vi "Start Logic-Mode dependent case 2.vi"(6 "Case name string":string, 8 "error in (no error)":errorcluster, 9 "cancelled":bool, 10 "UI queue":refnum<queue>, 11 "Acq. queue in":refnum<queue>) -> (0 "error out":errorcluster, 3 "Acq. queue out":refnum<queue>)   [LabVIEW 2017]
uses:
  Queue/Message Queue/Typedefs/Message Cluster.ctl
  Typedefs/Read Write Enum.ctl
  Typedefs/Top level VI states.ctl
  Global Variables/gl_UI Ctrl Refs.vi
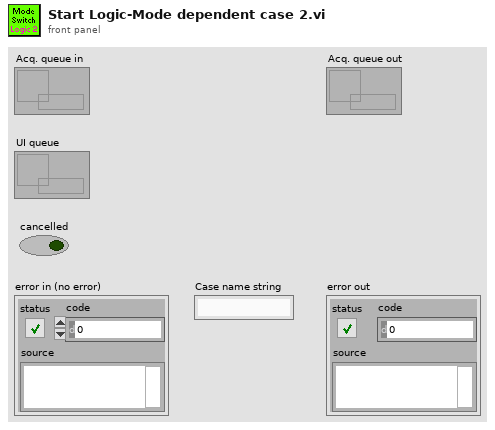
[diagram p1: front panel]
types:
  T1 = typedef "Read Write Enum.ctl" = enum16{"Read", "Write"}
  T2 = typedef "Top level VI states.ctl" = enum16{"None", "Initialise UI", "<STACK PROTOCOL STATES>", "AOL Zstack-START", "AOL Zstack-STOP", "Motor Zstack-START", "Motor Zstack-STOP", "<ACQUISITION PROTOCOL STATES> ", "Functional Acquisition-START", "Functional Acquisition-STOP", "Single Plane Acquisition-START", "Single Plane Acquisition-STOP", "Volume Acquisition-START", "Volume Acquisition-STOP", "<LIVE IMAGING PROTOCOL STATES>", "Live Imaging-START", "Live Imaging-STOP", "Live Plane Imaging-START", "Live Plane Imaging-STOP", "Live Volume Imaging-START", "Live Volume Imaging-STOP", "<MOVEMENT CORRECTION PROTOCOL STATES>", "EXIT"}
  T3 = typedef "UI ctrl refs cluster.ctl" = cluster{"Top level VI path":path, "Top level VI ref":refnum<vi>, "User menu ref":refnum<k9>, "Sub Panel control":refnum<vi>, "Imaging Param Tab":refnum<vi>, "Occurrence-Start drivers":refnum<k4>, "Occurrence-Speed logging initialised":refnum<k4>, "Occurrence-XYZ stage initialised":refnum<k4>, "Exit button":refnum<vi>, "Status ind":refnum<vi>, "Set as origin":refnum<vi>, "Speed Logging":refnum<vi>, "Time Lapse":refnum<vi>, "Live Imaging":refnum<vi>, "AOL Z Stack":refnum<vi>, "Motor Z Stack":refnum<vi>, "Funct Acq button":refnum<vi>, "Hard Shutter":refnum<vi>, "Virtual Shutter":refnum<vi>, "Laser Power":refnum<vi>, "AOL Mode":refnum<vi>, "Frame Size":refnum<vi>, "Field of View":refnum<vi>, "Dwell Time":refnum<vi>, "Zoom":refnum<vi>, "AOL Z":refnum<vi>, "Objective":refnum<vi>, "Axis":refnum<vi>, "Paths & Names":refnum<vi>, "Experiment folder path (ind.)":refnum<vi>, "Last State (Ind.)":refnum<vi>, "Averages":refnum<vi>, "Angle (degrees)":refnum<vi>, "X centre":refnum<vi>, "Y centre":refnum<vi>, "Plane Mode":refnum<vi>, "# Planes":refnum<vi>, "Z Start":refnum<vi>, "Z Stop":refnum<vi>, "Z Step":refnum<vi>, "PMT 1":refnum<vi>, "PMT 2":refnum<vi>, "Stage XYZ Position":refnum<vi>, "Pockels@Z Start":refnum<vi>, "Pockels@Z Stop":refnum<vi>, "Obtain Z Start":refnum<vi>, "Obtain Z Stop":refnum<vi>, "Live stim.trig.period":refnum<vi>, "Live stim.trig.enable":refnum<vi>, "XY Stage Move":refnum<vi>, "Funct. Acq. Pockels Modulation":refnum<vi>, "Enable Video Recording":refnum<vi>, "Video Record-Live Imaging":refnum<vi>, "Video Record-Funct acq":refnum<vi>, "AOL Z-stack Chirps Ready (ind)":refnum<vi>, "Target time between mov.cor. ref triggers (ms)":refnum<vi>, "Center freq ind (nm)":refnum<vi>, "Pickup mode (ind)":refnum<vi>, "Logging queue (ind)":refnum<vi>, "Back aperture power (ind.)":refnum<vi>, "Power after objective (ind.)":refnum<vi>, "Switch user":refnum<vi>, "Ls1 Conn. Status":refnum<vi>, "Ls1Tuning Status":refnum<vi>, "Ls1 Faults":refnum<vi>, "Ls1 Connection":refnum<vi>, "Ls1 Mode":refnum<vi>, "Ls1 POWER [mW]":refnum<vi>, "Ls1Shutter":refnum<vi>, "Ls1 Wavelength":refnum<vi>, "Ls1 Note":refnum<vi>, "Ls1 Confirm Wav":refnum<vi>, "Ls1 PreChrp Prism1":refnum<vi>, "Ls1 PreChrp Prism2":refnum<vi>, "Ls1 wav top Ind":refnum<vi>, "Ls1 power top Ind":refnum<vi>, "Ls1 Pump peak Hold":refnum<vi>, "Ls1 Status Ind":refnum<vi>, "Ls1 wav cancel":refnum<vi>, "Experiment Type":refnum<vi>, "Biology Information":refnum<vi>}
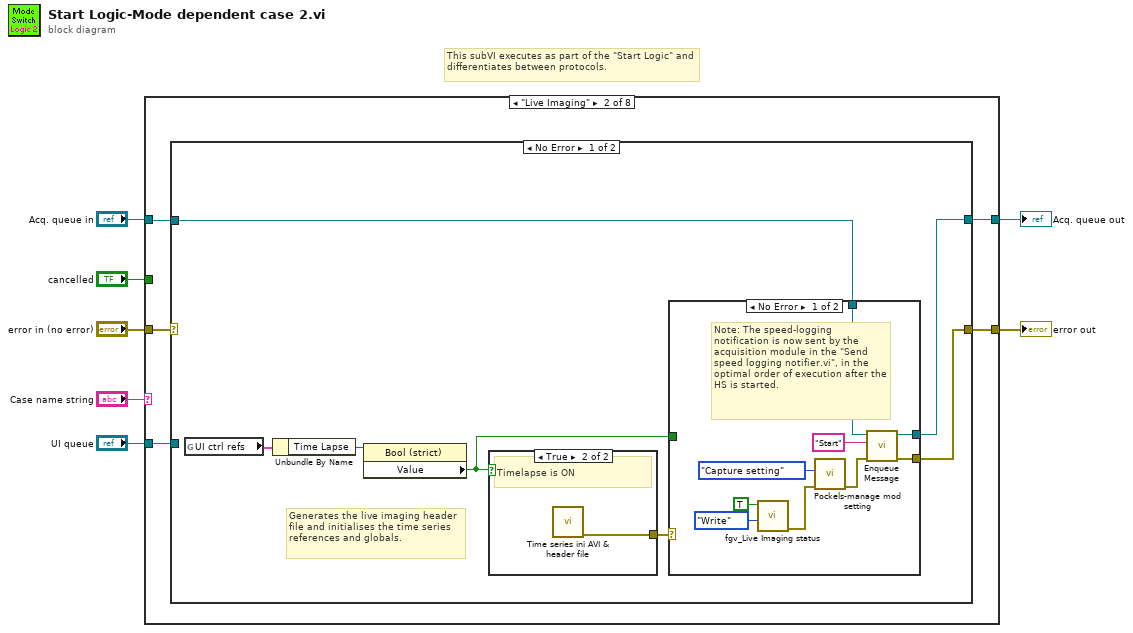
[diagram p0: block diagram]
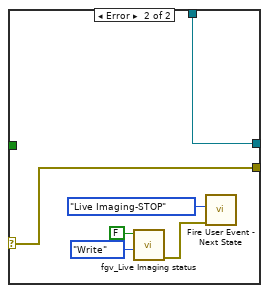
[diagram p3: hidden frame]
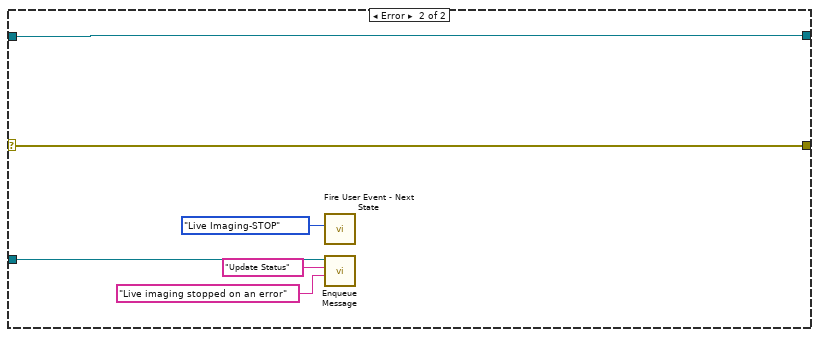
[diagram p5: hidden frame]
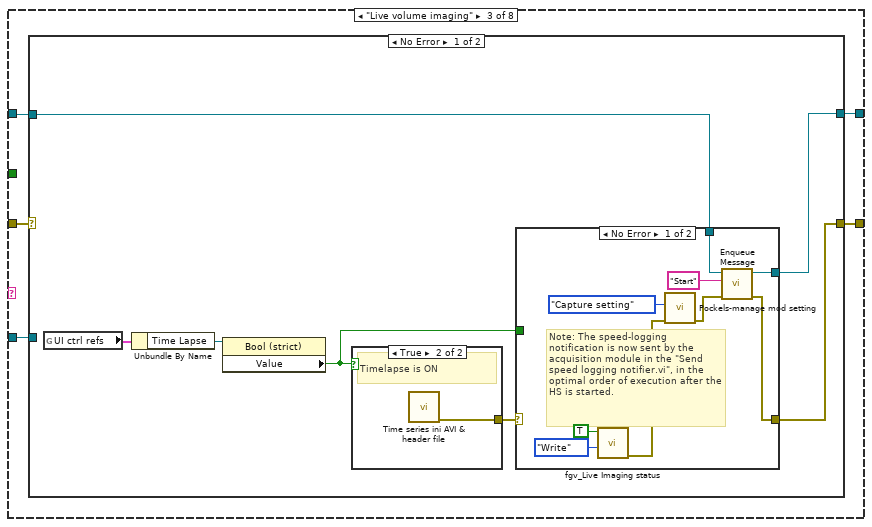
[diagram p6: hidden frame]
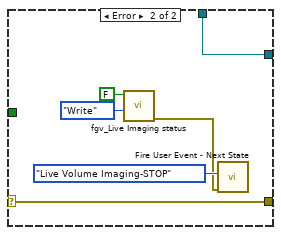
[diagram p7: hidden frame]
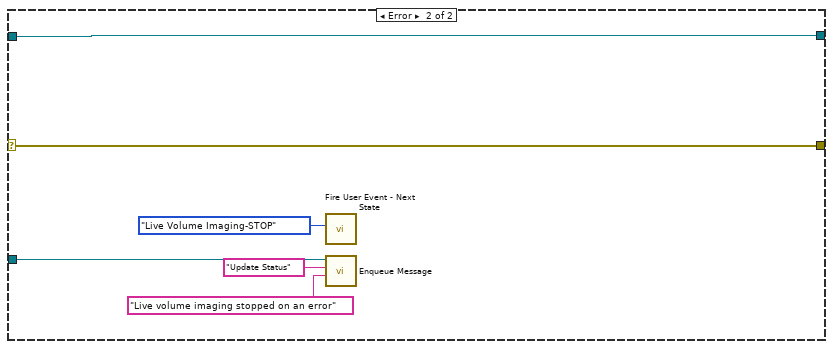
[diagram p9: hidden frame]
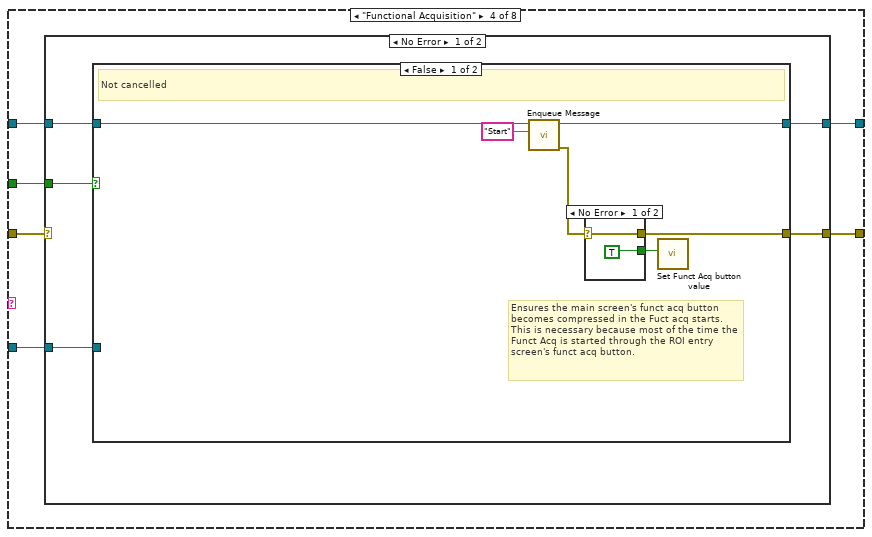
[diagram p10: hidden frame]
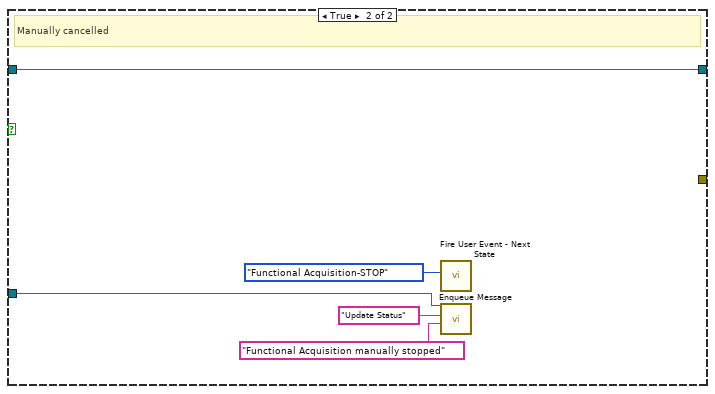
[diagram p12: hidden frame]
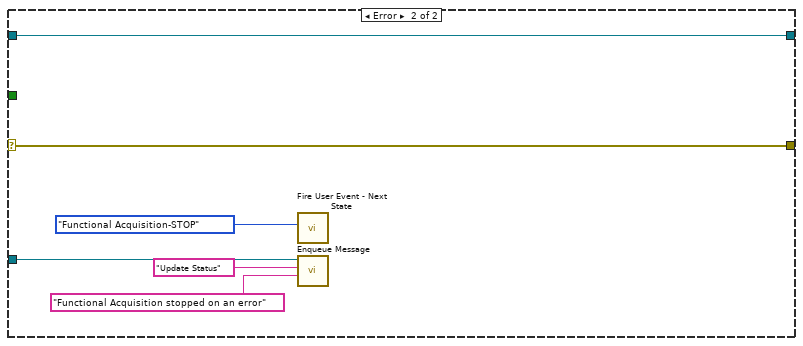
[diagram p13: hidden frame]
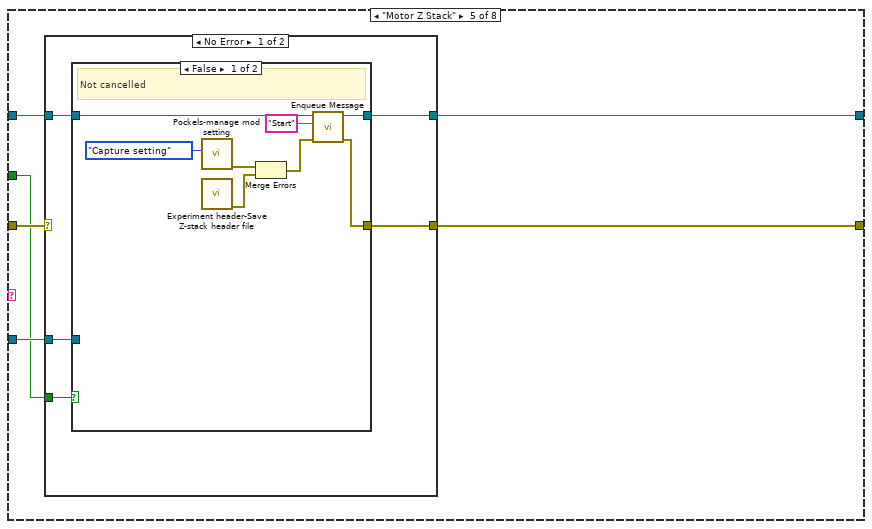
[diagram p14: hidden frame]
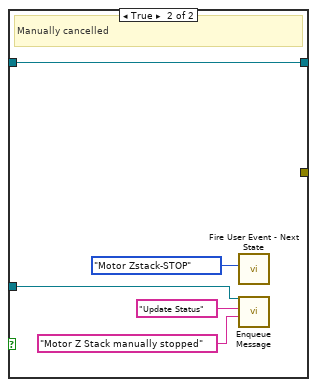
[diagram p15: hidden frame]
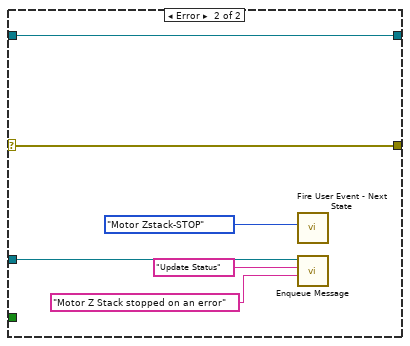
[diagram p16: hidden frame]
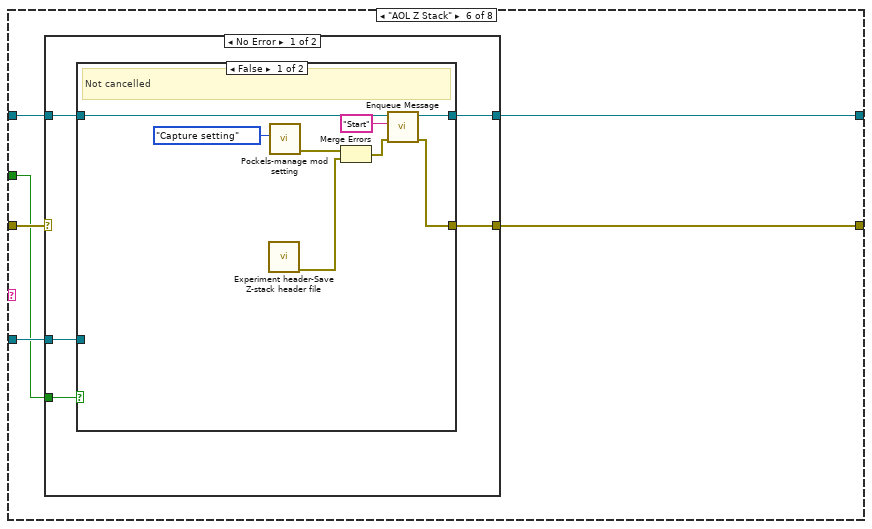
[diagram p17: hidden frame]
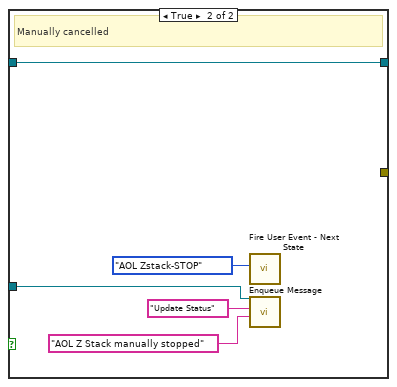
[diagram p18: hidden frame]
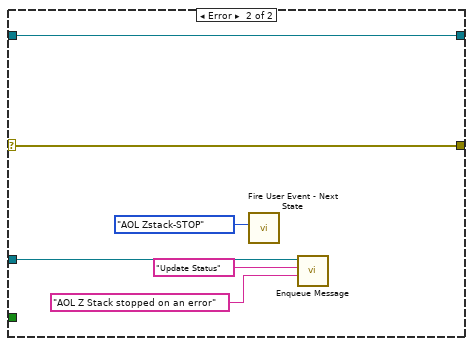
[diagram p19: hidden frame]
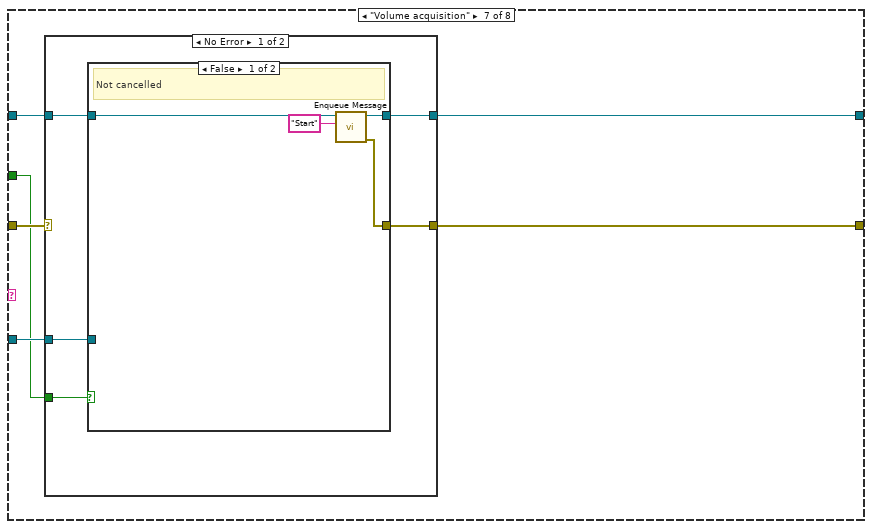
[diagram p20: hidden frame]
diagram:
  # "This subVI executes as part of the \"Start Logic\" and differentiates between protocols."
  n1 = case shown="\"Live Imaging\"" "Case name string" {
    tunnel: [w9 w14 w48 w80 w111 w141 w171 w197] -> w1
    tunnel: "error in (no error)" -> [w9 w11 w45 w81 w112 w142 w172 w198]
    tunnel: [w8 w12 w46 w83 w114 w144 w174 w200] -> w3
    tunnel: "Acq. queue in" -> [w8 w13 w47 w82 w113 w143 w173 w199]
    tunnel: "UI queue" -> [_ w10 w44 w79 w110 w140 w170 w196]
    tunnel: "cancelled" -> [_ _ _ w78 w109 w139 w169 w195]
    frame Default {
    }
    frame "Live Imaging" {
      n2 = case shown="No Error" w11 {
        selector: w11 -> [_ w43]
        tunnel: [w16 w43] -> w14
        tunnel: w13 -> [w18 w42]
        tunnel: [w17 w42] -> w12
        tunnel: w10 -> [_ w38]
        frame No Error {
          # "Generates the live imaging header file and initialises the time series references and globals."
          n3 = global read "gl_UI Ctrl Refs.vi" "UI ctrl refs"() -> (w15:T3)
          n4 = Unbundle By Name(w15) -> ("Time Lapse"=w21:refnum<vi>)
          n5 = property class="Bool (strict)"(reference=w21) -> ("Value"=w19:bool)  [unwired: 1 in, 2 out]
          n6 = case shown="True" w19 {
            tunnel: [_ w37] -> w20
            frame False {
              # "Timelapse is OFF"
            }
            frame True {
              # "Timelapse is ON"
              n7 = call "Time series ini AVI & header file.vi"() -> ("error out"=w37:errorcluster)  [unwired: 11 in]
            }
          }
          n8 = case shown="No Error" w20 {
            selector: w20 -> [_ w34]
            tunnel: w19 -> [_ _]
            tunnel: w18 -> [w27 w35]
            tunnel: [w29 w35] -> w17
            tunnel: [w28 w34] -> w16
            frame No Error {
              # "Note: The speed-logging notification is now sent by the acquisition module in the \"Send speed logging notifier.vi\", in the optimal order of execution after the HS is started."
              n9 = call "fgv_Live Imaging status.vi"("Function"=Read_Write_Enum."Write", "Live Imaging?"=TRUE ("Timelapse?")) -> ("error out"=w22:errorcluster)  [unwired: 8 in, 1 out]
              n10 = call "Pockels-manage mod setting.vi"("error in (no error)"=w22, "Function"=enum16{"Capture setting", "Re-apply setting"}."Capture setting") -> ("error out"=w26:errorcluster)  [unwired: 9 in]
              n11 = call "Enqueue Message.vi"("error in (no error)"=w26, "Message"="Start", "Queue"=w27) -> ("error out"=w28:errorcluster, "Queue out"=w29:refnum<queue>)  [unwired: 7 in]
            }
            frame Error {
              n12 = call "fgv_Live Imaging status.vi"("Function"=Read_Write_Enum."Write", "Live Imaging?"=FALSE ("Timelapse?")) -> ("error out"=w31:errorcluster)  [unwired: 8 in, 1 out]
              n13 = call "Fire User Event - Next State.vi"("Error In"=w31, "\"UI Handler loop\" case to execute"=Top_level_VI_states."Live Imaging-STOP" ("event data / imaging mode")) -> ()  [unwired: 9 in, 1 out]
            }
          }
        }
        frame Error {
          n14 = call "Fire User Event - Next State.vi"("\"UI Handler loop\" case to execute"=Top_level_VI_states."Live Imaging-STOP" ("event data / imaging mode")) -> ()  [unwired: 10 in, 1 out]
          n15 = call "Enqueue Message.vi"("Message Data"="Live imaging stopped on an error" ("Acquiring and Logging..."), "Message"="Update Status", "Queue"=w38) -> ()  [unwired: 7 in, 2 out]
        }
      }
    }
    frame "Live volume imaging" {
      n16 = case shown="No Error" w45 {
        selector: w45 -> [_ w77]
        tunnel: [w52 w77] -> w48
        tunnel: w47 -> [w51 w76]
        tunnel: [w50 w76] -> w46
        tunnel: w44 -> [_ w73]
        frame No Error {
          n17 = global read "gl_UI Ctrl Refs.vi" "UI ctrl refs"() -> (w49:T3)
          n18 = Unbundle By Name(w49) -> ("Time Lapse"=w55:refnum<vi>)
          n19 = property class="Bool (strict)"(reference=w55) -> ("Value"=w53:bool)  [unwired: 1 in, 2 out]
          n20 = case shown="True" w53 {
            tunnel: [_ w71] -> w54
            frame False {
              # "Timelapse is OFF"
            }
            frame True {
              # "Timelapse is ON"
              n21 = call "Time series ini AVI & header file.vi"() -> ("error out"=w71:errorcluster)  [unwired: 11 in]
            }
          }
          n22 = case shown="No Error" w54 {
            selector: w54 -> [_ w70]
            tunnel: [w63 w70] -> w52
            tunnel: w53 -> [_ _]
            tunnel: w51 -> [w62 w68]
            tunnel: [w61 w68] -> w50
            frame No Error {
              # "Note: The speed-logging notification is now sent by the acquisition module in the \"Send speed logging notifier.vi\", in the optimal order of execution after the HS is started."
              n23 = call "fgv_Live Imaging status.vi"("Function"=Read_Write_Enum."Write", "Live Imaging?"=TRUE ("Timelapse?")) -> ("error out"=w56:errorcluster)  [unwired: 8 in, 1 out]
              n24 = call "Pockels-manage mod setting.vi"("error in (no error)"=w56, "Function"=enum16{"Capture setting", "Re-apply setting"}."Capture setting") -> ("error out"=w60:errorcluster)  [unwired: 9 in]
              n25 = call "Enqueue Message.vi"("error in (no error)"=w60, "Message"="Start", "Queue"=w62) -> ("error out"=w63:errorcluster, "Queue out"=w61:refnum<queue>)  [unwired: 7 in]
            }
            frame Error {
              n26 = call "fgv_Live Imaging status.vi"("Function"=Read_Write_Enum."Write", "Live Imaging?"=FALSE ("Timelapse?")) -> ("error out"=w65:errorcluster)  [unwired: 8 in, 1 out]
              n27 = call "Fire User Event - Next State.vi"("Error In"=w65, "\"UI Handler loop\" case to execute"=Top_level_VI_states."Live Volume Imaging-STOP" ("event data / imaging mode")) -> ()  [unwired: 9 in, 1 out]
            }
          }
        }
        frame Error {
          n28 = call "Fire User Event - Next State.vi"("\"UI Handler loop\" case to execute"=Top_level_VI_states."Live Volume Imaging-STOP" ("event data / imaging mode")) -> ()  [unwired: 10 in, 1 out]
          n29 = call "Enqueue Message.vi"("Message Data"="Live volume imaging stopped on an error" ("Acquiring and Logging..."), "Message"="Update Status", "Queue"=w73) -> ()  [unwired: 7 in, 2 out]
        }
      }
    }
    frame "Functional Acquisition" {
      n30 = case shown="No Error" w81 {
        selector: w81 -> [_ w107]
        tunnel: [w84 w107] -> w80
        tunnel: [w85 w108] -> w83
        tunnel: w82 -> [w86 w108]
        tunnel: w79 -> [w88 w103]
        tunnel: w78 -> [w87 _]
        frame No Error {
          n31 = case shown="False" w87 {
            tunnel: w88 -> [_ w99]
            tunnel: w86 -> [w93 w98]
            tunnel: [w92 w98] -> w85
            tunnel: [w90 _] -> w84
            frame False {
              # "Ensures the main screen's funct acq button becomes compressed in the Fuct acq starts. This is necessary because most of the time the Funct Acq is started through the ROI entry screen's funct acq button."
              # "Not cancelled"
              n32 = call "Enqueue Message.vi"("Message"="Start", "Queue"=w93) -> ("error out"=w91:errorcluster, "Queue out"=w92:refnum<queue>)  [unwired: 8 in]
              n33 = case shown="No Error" w91 {
                selector: w91 -> [w96 w97]
                tunnel: [w96 w97] -> w90
                tunnel: [TRUE ("Value") _] -> w89
                frame No Error {
                }
                frame Error {
                }
              }
              n34 = call "Set Funct Acq button value.vi"("Functional Acquisition button's new value"=w89) -> ()  [unwired: 10 in, 1 out]
            }
            frame True {
              # "Manually cancelled"
              n35 = call "Fire User Event - Next State.vi"("\"UI Handler loop\" case to execute"=Top_level_VI_states."Functional Acquisition-STOP" ("event data / imaging mode")) -> ()  [unwired: 10 in, 1 out]
              n36 = call "Enqueue Message.vi"("Message Data"="Functional Acquisition manually stopped" ("Acquiring and Logging..."), "Message"="Update Status", "Queue"=w99) -> ()  [unwired: 7 in, 2 out]
            }
          }
        }
        frame Error {
          n37 = call "Fire User Event - Next State.vi"("\"UI Handler loop\" case to execute"=Top_level_VI_states."Functional Acquisition-STOP" ("event data / imaging mode")) -> ()  [unwired: 10 in, 1 out]
          n38 = call "Enqueue Message.vi"("Message Data"="Functional Acquisition stopped on an error" ("Acquiring and Logging..."), "Message"="Update Status", "Queue"=w103) -> ()  [unwired: 7 in, 2 out]
        }
      }
    }
    frame "Motor Z Stack" {
      n39 = case shown="No Error" w112 {
        selector: w112 -> [_ w137]
        tunnel: [w115 w137] -> w111
        tunnel: [w116 w138] -> w114
        tunnel: w113 -> [w117 w138]
        tunnel: w110 -> [w119 w133]
        tunnel: w109 -> [w118 _]
        frame No Error {
          n40 = case shown="False" w118 {
            tunnel: w119 -> [_ w129]
            tunnel: w117 -> [w126 w128]
            tunnel: [w125 w128] -> w116
            tunnel: [w124 _] -> w115
            frame False {
              # "Not cancelled"
              n41 = call "Pockels-manage mod setting.vi"("Function"=enum16{"Capture setting", "Re-apply setting"}."Capture setting") -> ("error out"=w122:errorcluster)  [unwired: 10 in]
              n42 = call "Experiment header-Save Z-stack header file.vi"() -> ("error out"=w121:errorcluster)  [unwired: 11 in]
              n43 = Merge Errors(w122, w121) -> (w120:errorcluster)
              n44 = call "Enqueue Message.vi"("error in (no error)"=w120, "Message"="Start", "Queue"=w126) -> ("error out"=w124:errorcluster, "Queue out"=w125:refnum<queue>)  [unwired: 7 in]
            }
            frame True {
              # "Manually cancelled"
              n45 = call "Fire User Event - Next State.vi"("\"UI Handler loop\" case to execute"=Top_level_VI_states."Motor Zstack-STOP" ("event data / imaging mode")) -> ()  [unwired: 10 in, 1 out]
              n46 = call "Enqueue Message.vi"("Message Data"="Motor Z Stack manually stopped" ("Acquiring and Logging..."), "Message"="Update Status", "Queue"=w129) -> ()  [unwired: 7 in, 2 out]
            }
          }
        }
        frame Error {
          n47 = call "Fire User Event - Next State.vi"("\"UI Handler loop\" case to execute"=Top_level_VI_states."Motor Zstack-STOP" ("event data / imaging mode")) -> ()  [unwired: 10 in, 1 out]
          n48 = call "Enqueue Message.vi"("Message Data"="Motor Z Stack stopped on an error" ("Acquiring and Logging..."), "Message"="Update Status", "Queue"=w133) -> ()  [unwired: 7 in, 2 out]
        }
      }
    }
    frame "AOL Z Stack" {
      n49 = case shown="No Error" w142 {
        selector: w142 -> [_ w167]
        tunnel: [w145 w167] -> w141
        tunnel: [w146 w168] -> w144
        tunnel: w143 -> [w147 w168]
        tunnel: w140 -> [w149 w163]
        tunnel: w139 -> [w148 _]
        frame No Error {
          n50 = case shown="False" w148 {
            tunnel: w149 -> [_ w159]
            tunnel: w147 -> [w156 w158]
            tunnel: [w155 w158] -> w146
            tunnel: [w154 _] -> w145
            frame False {
              # "Not cancelled"
              n51 = call "Experiment header-Save Z-stack header file.vi"() -> ("error out"=w150:errorcluster)  [unwired: 11 in]
              n52 = call "Pockels-manage mod setting.vi"("Function"=enum16{"Capture setting", "Re-apply setting"}."Capture setting") -> ("error out"=w152:errorcluster)  [unwired: 10 in]
              n53 = Merge Errors(w152, w150) -> (w151:errorcluster)
              n54 = call "Enqueue Message.vi"("error in (no error)"=w151, "Message"="Start", "Queue"=w156) -> ("error out"=w154:errorcluster, "Queue out"=w155:refnum<queue>)  [unwired: 7 in]
            }
            frame True {
              # "Manually cancelled"
              n55 = call "Fire User Event - Next State.vi"("\"UI Handler loop\" case to execute"=Top_level_VI_states."AOL Zstack-STOP" ("event data / imaging mode")) -> ()  [unwired: 10 in, 1 out]
              n56 = call "Enqueue Message.vi"("Message Data"="AOL Z Stack manually stopped" ("Acquiring and Logging..."), "Message"="Update Status", "Queue"=w159) -> ()  [unwired: 7 in, 2 out]
            }
          }
        }
        frame Error {
          n57 = call "Fire User Event - Next State.vi"("\"UI Handler loop\" case to execute"=Top_level_VI_states."AOL Zstack-STOP" ("event data / imaging mode")) -> ()  [unwired: 10 in, 1 out]
          n58 = call "Enqueue Message.vi"("Message Data"="AOL Z Stack stopped on an error" ("Acquiring and Logging..."), "Message"="Update Status", "Queue"=w163) -> ()  [unwired: 7 in, 2 out]
        }
      }
    }
    frame "Volume acquisition" {
      n59 = case shown="No Error" w172 {
        selector: w172 -> [_ w193]
        tunnel: [w175 w193] -> w171
        tunnel: [w176 w194] -> w174
        tunnel: w173 -> [w177 w194]
        tunnel: w170 -> [w179 w189]
        tunnel: w169 -> [w178 _]
        frame No Error {
          n60 = case shown="False" w178 {
            tunnel: w179 -> [_ w185]
            tunnel: w177 -> [w182 w184]
            tunnel: [w181 w184] -> w176
            tunnel: [w180 _] -> w175
            frame False {
              # "Not cancelled"
              n61 = call "Enqueue Message.vi"("Message"="Start", "Queue"=w182) -> ("error out"=w180:errorcluster, "Queue out"=w181:refnum<queue>)  [unwired: 8 in]
            }
            frame True {
              # "Manually cancelled"
              n62 = call "Fire User Event - Next State.vi"("\"UI Handler loop\" case to execute"=Top_level_VI_states."Volume Acquisition-STOP" ("event data / imaging mode")) -> ()  [unwired: 10 in, 1 out]
              n63 = call "Enqueue Message.vi"("Message Data"="Volume Acquisition manually stopped" ("Acquiring and Logging..."), "Message"="Update Status", "Queue"=w185) -> ()  [unwired: 7 in, 2 out]
            }
          }
        }
        frame Error {
          n64 = call "Fire User Event - Next State.vi"("\"UI Handler loop\" case to execute"=Top_level_VI_states."Volume Acquisition-STOP" ("event data / imaging mode")) -> ()  [unwired: 10 in, 1 out]
          n65 = call "Enqueue Message.vi"("Message Data"="Volume Acquisition stopped on an error" ("Acquiring and Logging..."), "Message"="Update Status", "Queue"=w189) -> ()  [unwired: 7 in, 2 out]
        }
      }
    }
    frame "Single Plane Acquisition" {
      n66 = case shown="No Error" w198 {
        selector: w198 -> [_ w222]
        tunnel: [w201 w222] -> w197
        tunnel: [w202 w223] -> w200
        tunnel: w199 -> [w203 w223]
        tunnel: w196 -> [w205 w218]
        tunnel: w195 -> [w204 _]
        frame No Error {
          n67 = case shown="False" w204 {
            tunnel: w205 -> [_ w214]
            tunnel: w203 -> [w211 w213]
            tunnel: [w210 w213] -> w202
            tunnel: [w209 _] -> w201
            frame False {
              # "Not cancelled"
              n68 = call "Pockels-manage mod setting.vi"("Function"=enum16{"Capture setting", "Re-apply setting"}."Capture setting") -> ("error out"=w207:errorcluster)  [unwired: 10 in]
              n69 = Merge Errors(w207) -> (w206:errorcluster)
              n70 = call "Enqueue Message.vi"("error in (no error)"=w206, "Message"="Start", "Queue"=w211) -> ("error out"=w209:errorcluster, "Queue out"=w210:refnum<queue>)  [unwired: 7 in]
            }
            frame True {
              # "Manually cancelled"
              n71 = call "Fire User Event - Next State.vi"("\"UI Handler loop\" case to execute"=Top_level_VI_states."Single Plane Acquisition-STOP" ("event data / imaging mode")) -> ()  [unwired: 10 in, 1 out]
              n72 = call "Enqueue Message.vi"("Message Data"="Single Plane Acquisition manually stopped" ("Acquiring and Logging..."), "Message"="Update Status", "Queue"=w214) -> ()  [unwired: 7 in, 2 out]
            }
          }
        }
        frame Error {
          n73 = call "Fire User Event - Next State.vi"("\"UI Handler loop\" case to execute"=Top_level_VI_states."Single Plane Acquisition-STOP" ("event data / imaging mode")) -> ()  [unwired: 10 in, 1 out]
          n74 = call "Enqueue Message.vi"("Message Data"="Single Plane Acquisition stopped on an error" ("Acquiring and Logging..."), "Message"="Update Status", "Queue"=w218) -> ()  [unwired: 7 in, 2 out]
        }
      }
    }
  }
  "Acq. queue out" <- w3
  "error out" <- w1
